vi "abortDriver_Feng_MFP3D.vi"(10 "litho comm":T2) -> ()   [LabVIEW 2016]
uses:
  <userlib>/LevyLab/Relay Box/Type_defs/Resistor--enum.ctl
  Driver Variables_MFP3D.vi
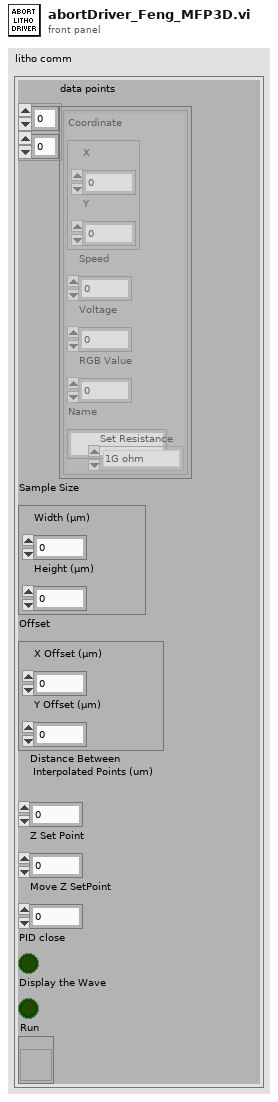
[diagram p1: front panel]
types:
  T1 = typedef "Resistor--enum.ctl" = enum16{"open", "discharge tip", "0 ohms", "100k ohm", "10M ohm", "1G ohm"}
  T2 = cluster{"data points":cluster{"Coordinate":cluster{"X":dbl, "Y":dbl}, "Speed":dbl, "Voltage":dbl, "RGB Value":i32, "Name":string, "Set Resistance":T1}[][], "Sample Size":cluster{"Width (µm)":dbl, "Height (µm)":dbl}, "Offset":cluster{"X Offset (µm)":dbl, "Y Offset (µm)":dbl}, "Distance Between\n Interpolated Points (um)":dbl, "Z Set Point":dbl, "Move Z SetPoint":dbl, "PID close":bool, "Display the Wave":bool, "Run":refnum<vi>}
  T3 = cluster{"Coordinate":cluster{"X":dbl, "Y":dbl}, "Speed":dbl, "Voltage":dbl, "RGB Value":i32, "Name":string, "Set Resistance":T1}[][]
  T4 = cluster{"X Offset (µm)":dbl, "Y Offset (µm)":dbl}
  T5 = enum16{"open", "discharge tip", "0 ohms", "100k ohm", "10M ohm", "1G ohm"}
  T6 = cluster{"Coordinate":cluster{"X":dbl, "Y":dbl}, "Speed":dbl, "Voltage":dbl, "RGB Value":i32, "Name":string, "Set Resistance":T1}
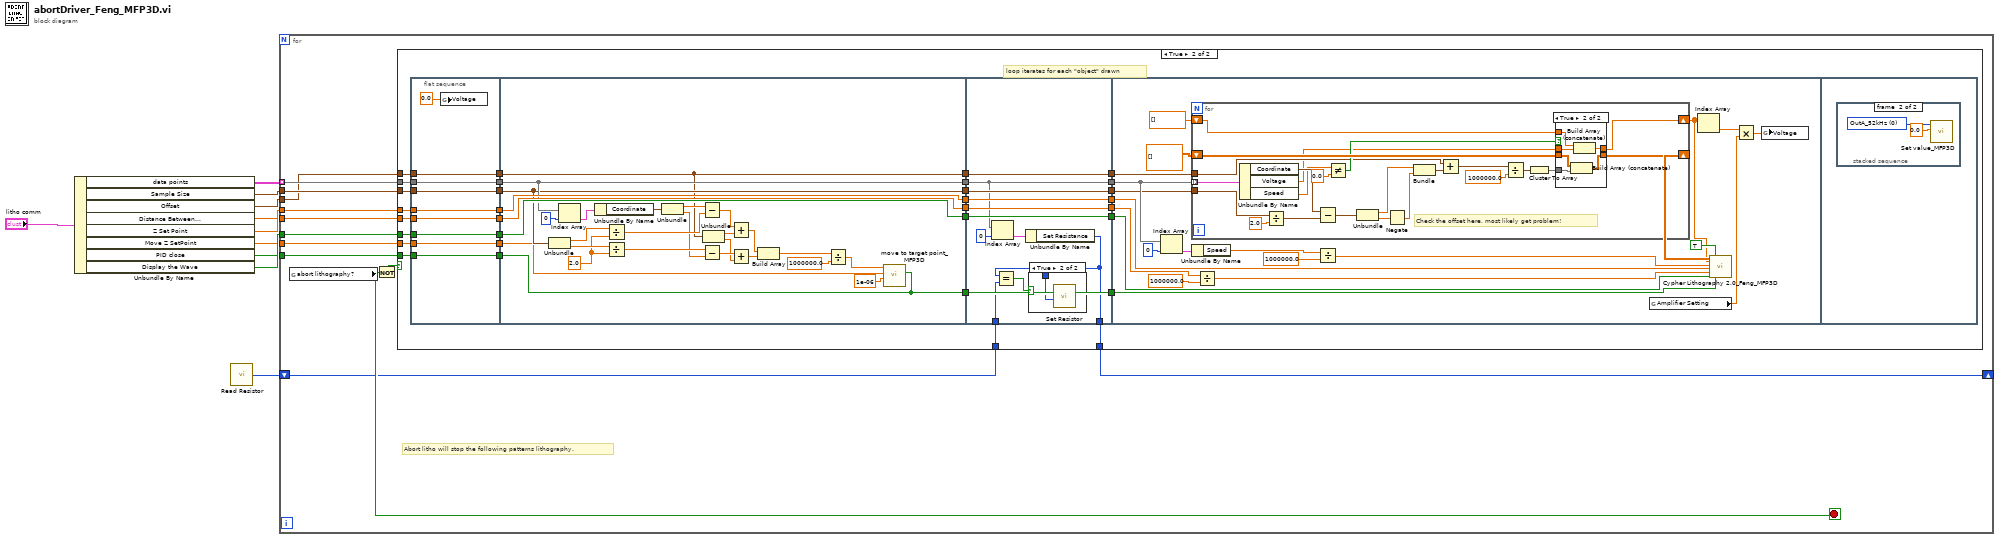
[diagram p0: block diagram]
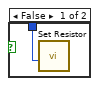
[diagram p3: hidden frame]
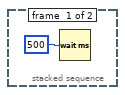
[diagram p5: hidden frame]
diagram:
  n1 = Unbundle By Name("litho comm") -> ("data points"=w3:T3, "Sample Size"=w4:cluster{"Width (µm)":dbl, "Height (µm)":dbl}, "Offset"=w5:T4, "Distance Between\n Interpolated Points (um)"=w6:dbl, "Z Set Point"=w7:dbl, "Move Z SetPoint"=w8:dbl, "PID close"=w9:bool, "Display the Wave"=w10:bool)
  n2 = call <userlib>:"Read Resistor.vi"() -> ("Set Resistance"=w1:T5)  [unwired: 1 in]
  n3 = for {
    tunnel: w6 -> [w17]
    tunnel: w3 -> [w22] mode=indexing
    tunnel: w7 -> [w21]
    tunnel: w10 -> [w20]
    tunnel: w9 -> [w19]
    tunnel: w4 -> [w18]
    tunnel: w5 -> [w16]
    tunnel: w8 -> [w15]
    shift-right: [w11] -> _
    shift-left: w1 -> [w12]
    stop <- w13 stop-if-true
    # "Abort litho will stop the following patterns lithography."
    n4 = global read "Driver Variables_MFP3D.vi" "abort lithography?"() -> (w13:bool)
    n5 = Not(x=w13) -> (.not. x?=w14:bool)
    n6 = case shown="True" w14 {
      tunnel: w22 -> [_ w47]
      tunnel: w21 -> [_ w46]
      tunnel: w20 -> [_ w45]
      tunnel: w19 -> [_ w44]
      tunnel: w18 -> [_ w43]
      tunnel: w17 -> [_ w42]
      tunnel: w16 -> [_ w41]
      tunnel: w15 -> [_ w40]
      tunnel: w12 -> [w23 w25]
      tunnel: [w23 w24] -> w11
      frame False {
      }
      frame True {
        # "loop iterates for each \"object\" drawn"
        n7 = flat-sequence {
          tunnel: w41 -> [w58]
          tunnel: w42 -> [w59]
          tunnel: w43 -> [w60]
          tunnel: w44 -> [w61]
          tunnel: w45 -> [w62]
          tunnel: w46 -> [w63]
          tunnel: w47 -> [w64]
          tunnel: [w64] -> w55
          tunnel: [w63] -> w54
          tunnel: [w62] -> w53
          tunnel: [w61] -> w52
          tunnel: [w60] -> w51
          tunnel: [w59] -> w50
          tunnel: [w58] -> w49
          tunnel: [w56] -> w48
          tunnel: w40 -> [w56]
          tunnel: [w69] -> w39
          tunnel: [w92] -> w37
          tunnel: [w91] -> w35
          tunnel: [w66] -> w33
          tunnel: [w68] -> w31
          tunnel: [w90] -> w29
          tunnel: [w67] -> w27
          tunnel: w55 -> [w69]
          tunnel: w54 -> [w92]
          tunnel: w53 -> [w91]
          tunnel: w52 -> [w66]
          tunnel: w51 -> [w68]
          tunnel: w50 -> [w90]
          tunnel: w49 -> [w67]
          tunnel: w48 -> [w65]
          tunnel: w39 -> [w97]
          tunnel: [w97] -> w38
          tunnel: w37 -> [w104]
          tunnel: [w104] -> w36
          tunnel: w35 -> [w103]
          tunnel: [w103] -> w34
          tunnel: w33 -> [w102]
          tunnel: [w102] -> w32
          tunnel: w31 -> [w101]
          tunnel: [w101] -> w30
          tunnel: w29 -> [w100]
          tunnel: [w100] -> w28
          tunnel: w27 -> [w99]
          tunnel: [w99] -> w26
          tunnel: w25 -> [w95]
          tunnel: [w93] -> w24
          tunnel: w38 -> [w128]
          tunnel: w36 -> [w113]
          tunnel: w34 -> [w115]
          tunnel: w32 -> [w116]
          tunnel: w30 -> [w125]
          tunnel: w28 -> [w121]
          tunnel: w26 -> [w119]
          frame #0 {
            n8 = global write "Driver Variables_MFP3D.vi" "Voltage"(0.0 ("Voltage")) -> ()
          }
          frame #1 {
            w81 = 2.0 ("y")
            n9 = Unbundle(w68) -> ("Width (µm)"=w85:dbl, "Height (µm)"=w82:dbl)
            n10 = Index Array(array=w69, index=0 ("index (row)")) -> (element=w88:T6)
            n11 = Unbundle By Name(w88) -> ("Coordinate"=w86:cluster{"X":dbl, "Y":dbl})
            n12 = Divide(x=w85, y=w81) -> (x/y=w83:dbl)
            n13 = Divide(x=w82, y=w81) -> (x/y=w80:dbl)
            n14 = Unbundle(w86) -> ("X"=w84:dbl, "Y"=w79:dbl)
            n15 = Subtract(x=w84, y=w83) -> (x-y=w78:dbl)
            n16 = Subtract(x=w80, y=w79) -> (x-y=w76:dbl)
            n17 = Unbundle(w67) -> ("X Offset (µm)"=w77:dbl, "Y Offset (µm)"=w75:dbl)
            n18 = Add(x=w78, y=w77) -> (x+y=w74:dbl)
            n19 = Add(x=w76, y=w75) -> (x+y=w73:dbl)
            n20 = Build Array(w74, w73) -> (w71:dbl[])
            n21 = Divide(x=w71, y=1000000.0) -> (x/y=w70:dbl[])
            n22 = call "move to target point_MFP3D.vi"("PIS Close"=w66, "Litho Speed"=1e-06, "Z SetPoint"=w65, "Target Point\n(  x      ,       y   )"=w70) -> ()  [unwired: 8 in]
          }
          frame #2 {
            n23 = Index Array(array=w97, index=0) -> (element=w96:T6)
            n24 = Unbundle By Name(w96) -> ("Set Resistance"=w93:T1)
            n25 = Equal?(x=w93, y=w95) -> (x = y?=w94:bool)
            n26 = case shown="True" w94 {
              tunnel: w93 -> [w105 w106]
              frame False {
                n27 = call <userlib>:"Set Resistor.vi"("Set Resistance"=w105) -> ()  [unwired: 10 in, 1 out]
              }
              frame True {
                n28 = call <userlib>:"Set Resistor.vi"("Set Resistance"=w106) -> ()  [unwired: 10 in, 1 out]
              }
            }
          }
          frame #3 {
            n29 = Index Array(array=w128, index=0) -> (element=w126:T6)
            n30 = for {
              tunnel: w128 -> [w151] mode=indexing
              tunnel: w125 -> [w149]
              shift-right: [w139] -> w111
              shift-left: dbl[][] [] -> [w138]
              tunnel: w119 -> [w132]
              shift-right: [w130] -> w109
              shift-left: dbl[] [] -> [w129]
              # "Check the offset here, most likely get problem!"
              n31 = Unbundle By Name(w151) -> ("Coordinate"=w146:cluster{"X":dbl, "Y":dbl}, "Voltage"=w131:dbl, "Speed"=w137:dbl)
              n32 = Divide(x=w149, y=2.0) -> (x/y=w145:cluster{"Width (µm)":dbl, "Height (µm)":dbl})
              n33 = Subtract(x=w146, y=w145) -> (x-y=w144:cluster{dbl, dbl})
              n34 = Not Equal?(x=w137, y=0.0) -> (x != y?=w135:bool)
              n35 = Unbundle(w144) -> (w141:dbl, w143:dbl)
              n36 = Negate(x=w143) -> (-x=w142:dbl)
              n37 = Bundle(w141, w142) -> (w134:cluster{dbl, dbl})  [unwired: 1 in]
              n38 = Add(x=w132, y=w134) -> (x+y=w133:cluster{dbl, dbl})
              n39 = Divide(x=w133, y=1000000.0) -> (x/y=w147:cluster{dbl, dbl})
              n40 = Cluster To Array(cluster=w147) -> (array=w140:dbl[])
              n41 = case shown="True" w135 {
                tunnel: w140 -> [_ w159]
                tunnel: [w153 w158] -> w139
                tunnel: w138 -> [w153 w157]
                tunnel: w131 -> [_ w156]
                tunnel: [w152 w155] -> w130
                tunnel: w129 -> [w152 w154]
                frame False {
                }
                frame True {
                  n42 = Build Array (concatenate)(w157, w159) -> (w158:dbl[][])
                  n43 = Build Array (concatenate)(w154, w156) -> (w155:dbl[])
                }
              }
            }
            n44 = Unbundle By Name(w126) -> ("Speed"=w123:dbl)
            n45 = Divide(x=w121, y=1000000.0) -> (x/y=w114:dbl)
            n46 = Divide(x=w123, y=1000000.0) -> (x/y=w112:dbl)
            n47 = global read "Driver Variables_MFP3D.vi" "Amplifier Setting"() -> (w118:dbl)
            n48 = Index Array(array=w109) -> (element=w117:dbl)  [unwired: 1 in]
            n49 = call "Cypher Lithography 2.0_Feng_MFP3D.vi"("Nodes on the line\n(  x      ,       y   )"=w111, "V"=w109, "Litho Speed"=w112, "Z SetPoint"=w113, "New nodes spacing"=w114, "display wave"=w115, "Need interpolate new nodes?"=TRUE, "PID close"=w116) -> ()  [unwired: 12 in]
            n50 = Multiply(x=w117, y=w118) -> (x*y=w108:dbl)
            n51 = global write "Driver Variables_MFP3D.vi" "Voltage"(w108) -> ()
          }
          frame #4 {
            n52 = stacked-sequence {
              frame #0 {
                n53 = Wait (ms)(milliseconds to wait=u32 500) -> ()  [unwired: 1 out]
              }
              frame #1 {
                w162 = u16 0 items=["OutA_52kHz", "OutB_52kHz", "OutC_78Hz", "PiezoX", "PiezoY", "PiezoZ", "DDS_Frequency1", "DDS_Frequency2", "DDS_Amplitude1", "DDS_Amplitude2", "DDS_DCOffset", "\"Setpoint%PIDSLoop.3\"", "\"Setpoint%PIDSLoop.4\"", ""] ("Output")
                n54 = call "Set value_MFP3D.vi"("Value"=0.0, "Output"=w162) -> ()  [unwired: 9 in, 1 out]
              }
            }
          }
        }
      }
    }
  }
